vi "ln.vi"(8 "ready for output (T)":bool=TRUE, 9 "input valid":bool, 10 "x":fxp<+/-,64,32>) -> (0 "ready for input":bool, 1 "output valid":bool, 2 "ln(x)":fxp<+/-,32,16>)   [LabVIEW 2018]
uses:
  <vilib>/rvi/FXPMathLib/FxpLn/subVIs/nifxpmath_NaturalLogarithm_SimConfig.ctl
  <vilib>/rvi/FXPMathLib/FxpLn/simVIs/DllFxpNaturalLogarithmTemp_sub.vi
  <vilib>/rvi/FXPMathLib/FxpMul/XNode/nifxpmath_Multiplier.xnode
  <vilib>/rvi/FXPMathLib/FxpLn/XNode/nifxpmath_NaturalLogarithm.xnode
  <vilib>/rvi/FXPMathLib/FxpAdd/XNode/nifxpmath_Add.xnode
  <vilib>/rvi/FXPMathLib/sim/FxpSim.dll
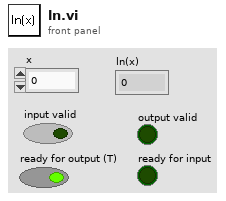
[diagram p1: front panel]
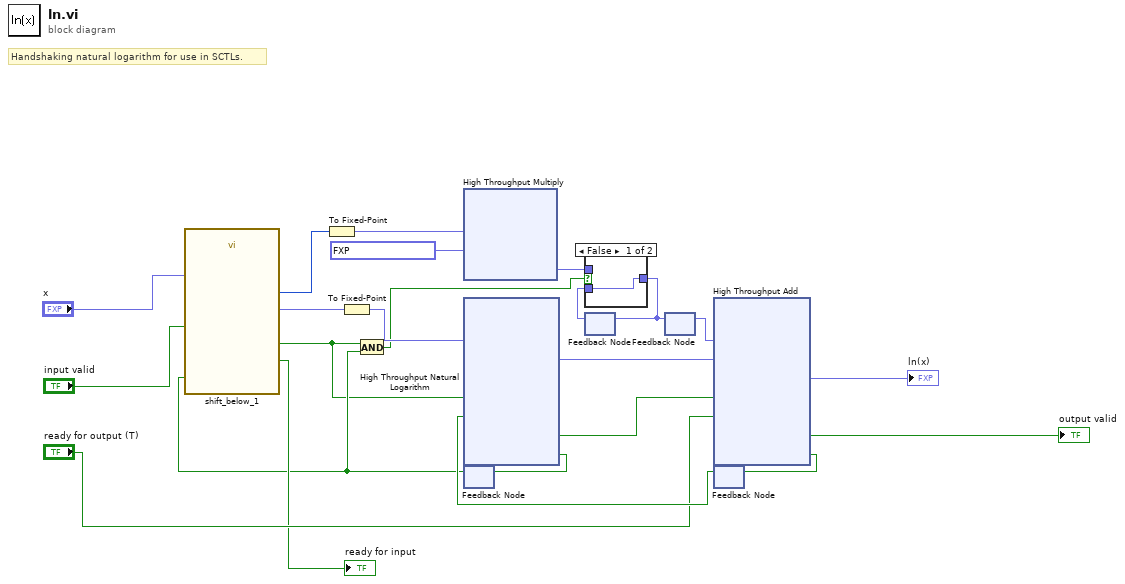
[diagram p0: block diagram]
diagram:
  # "Handshaking natural logarithm for use in SCTLs."
  n1 = feedback #1() -> (w6:bool)  [unwired: 1 in]
  n2 = call "shift_below_1.vi"("ready for output"=w6, "input valid"="input valid", "input"="x") -> ("ready for input"=→"ready for input":bool, "output valid"=w5:bool, "shifted"=w22:fxp<+/-,64,32>, "count"=w16:i16)  [unwired: 1 in]
  n3 = To Fixed-Point(number=w16) -> (fixed-point=w14:fxp<+/-,9,9>)  [unwired: 1 in]
  n4 = To Fixed-Point(number=w22) -> (fixed-point=w21:fxp<+,16,0>)  [unwired: 1 in]
  n5 = And(x=w5, y=w6) -> (x .and. y?=w4:bool)
  n6 = xnode "High Throughput Multiply"("x"=w14, "y"=fxp<+,32,16> 0.693145751953125) -> ("x*y"=w3:fxp<+/-,41,25>)
  n7 = feedback #2() -> (w2:fxp<+/-,41,25>)  [unwired: 1 in]
  n8 = case shown="False" w4 {
    tunnel: w3 -> [_ w25]
    tunnel: w2 -> [w24 _]
    tunnel: [w24 w25] -> w1
    frame False {
    }
    frame True {
    }
  }
  n9 = feedback-in #2(w1) -> ()
  n10 = feedback-in #3(w1) -> ()
  n11 = feedback #3() -> (w10:fxp<+/-,41,25>)  [unwired: 1 in]
  n12 = feedback #4() -> (w13:bool)  [unwired: 1 in]
  n13 = xnode "High Throughput Natural Logarithm"("x"=w21, "input valid"=w5, "ready for output (T)"=w13) -> ("ln(x)"=w17:fxp<+/-,16,1>, "output valid"=w8:bool, "ready for input"=w11:bool)  [unwired: 1 out]
  n14 = feedback-in #1(w11) -> ()
  n15 = xnode "High Throughput Add"("x"=w10, "y"=w17, "input valid"=w8, "ready for output (T)"="ready for output (T)") -> ("x+y"=→"ln(x)":fxp<+/-,42,26>, "output valid"=→"output valid":bool, "ready for input"=w18:bool)
  n16 = feedback-in #4(w18) -> ()
